vi "Get Table Values (VAR).vi"(7 "Sheet Name":string, 8 "error in":errorcluster, 10 "Table Name":string, 11 "SpreadsheetDoc in":refnum<k24>) -> (0 "error out":errorcluster, 2 "Cell Values":variant[][](array[variant]), 3 "SpreadsheetDoc out":refnum<k24>)   [LabVIEW 2019, in "Open Xml.lvlib"]
uses:
  Open Xml.lvlib
  D:/git/Open-Xml-LabVIEW/Source/DocumentFormat.OpenXml.dll
  DocumentFormat.OpenXml.dll
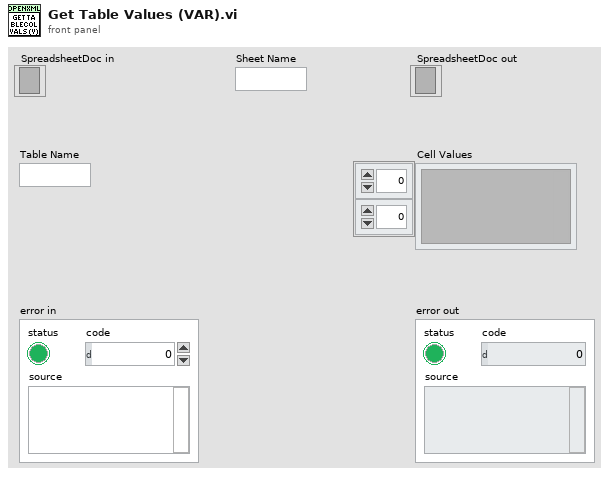
[diagram p1: front panel]
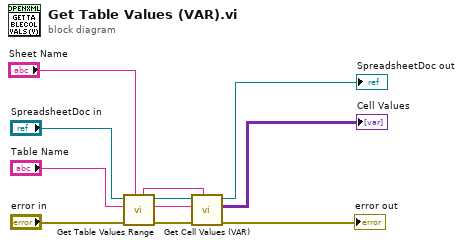
[diagram p0: block diagram]
diagram:
  n1 = call "Get Table Values Range.vi"("Sheet Name in"="Sheet Name", "error in"="error in", "Table Name"="Table Name", "SpreadsheetDoc in"="SpreadsheetDoc in") -> ("error out"=w4:errorcluster, "Range"=w2:string, "SpreadsheetDoc out"=w3:refnum<k24>, "Sheet Name out"=w1:string)  [unwired: 4 in]
  n2 = call "Get Cell Values (VAR).vi"("Sheet Name in"=w1, "error in"=w4, "Cell Range"=w2, "SpreadsheetDoc in"=w3) -> ("error out"=→"error out":errorcluster, "Cell Values"=→"Cell Values":variant[][], "SpreadsheetDoc out"=→"SpreadsheetDoc out":refnum<k24>)  [unwired: 5 in]
